vi "seatLeakageTest.vi"(7 "LabVIEW Web Service Request":refnum<class "Web Request.lvclass">, 10 "testPressure":dbl, 11 "time":dbl) -> (2 "startingPressure":dbl format="%#_2g", 3 "finalPressure":dbl)   [LabVIEW 2015]
uses:
  <vilib>/wsapi/Web Request.lvclass
  <vilib>/Waveform/WDTOps.llb/WDT Append Waveforms DBL.vi
panel:
  in  "Stop (Pressure Reading)":bool
  out "data":waveform(dbl)[](graph)
  out "timer":dbl
  in  "Stop timer":bool
  in  "Start timer":bool
  out "value":string
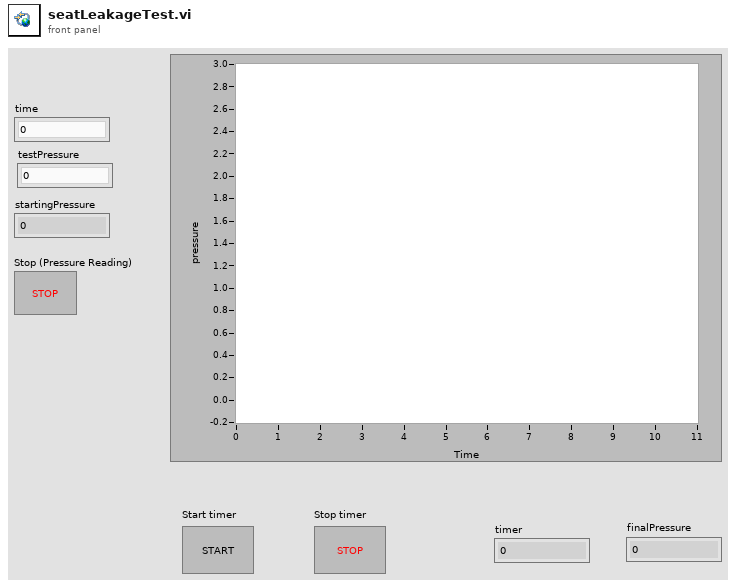
[diagram p1: front panel]
types:
  T1 = typedef "imagedata.ctl" = cluster{"image type":i32, "image depth":i32, "image":u8[], "mask":u8[], "colors":u32[], "Rectangle":cluster{"left":i16, "top":i16, "right":i16, "bottom":i16}}
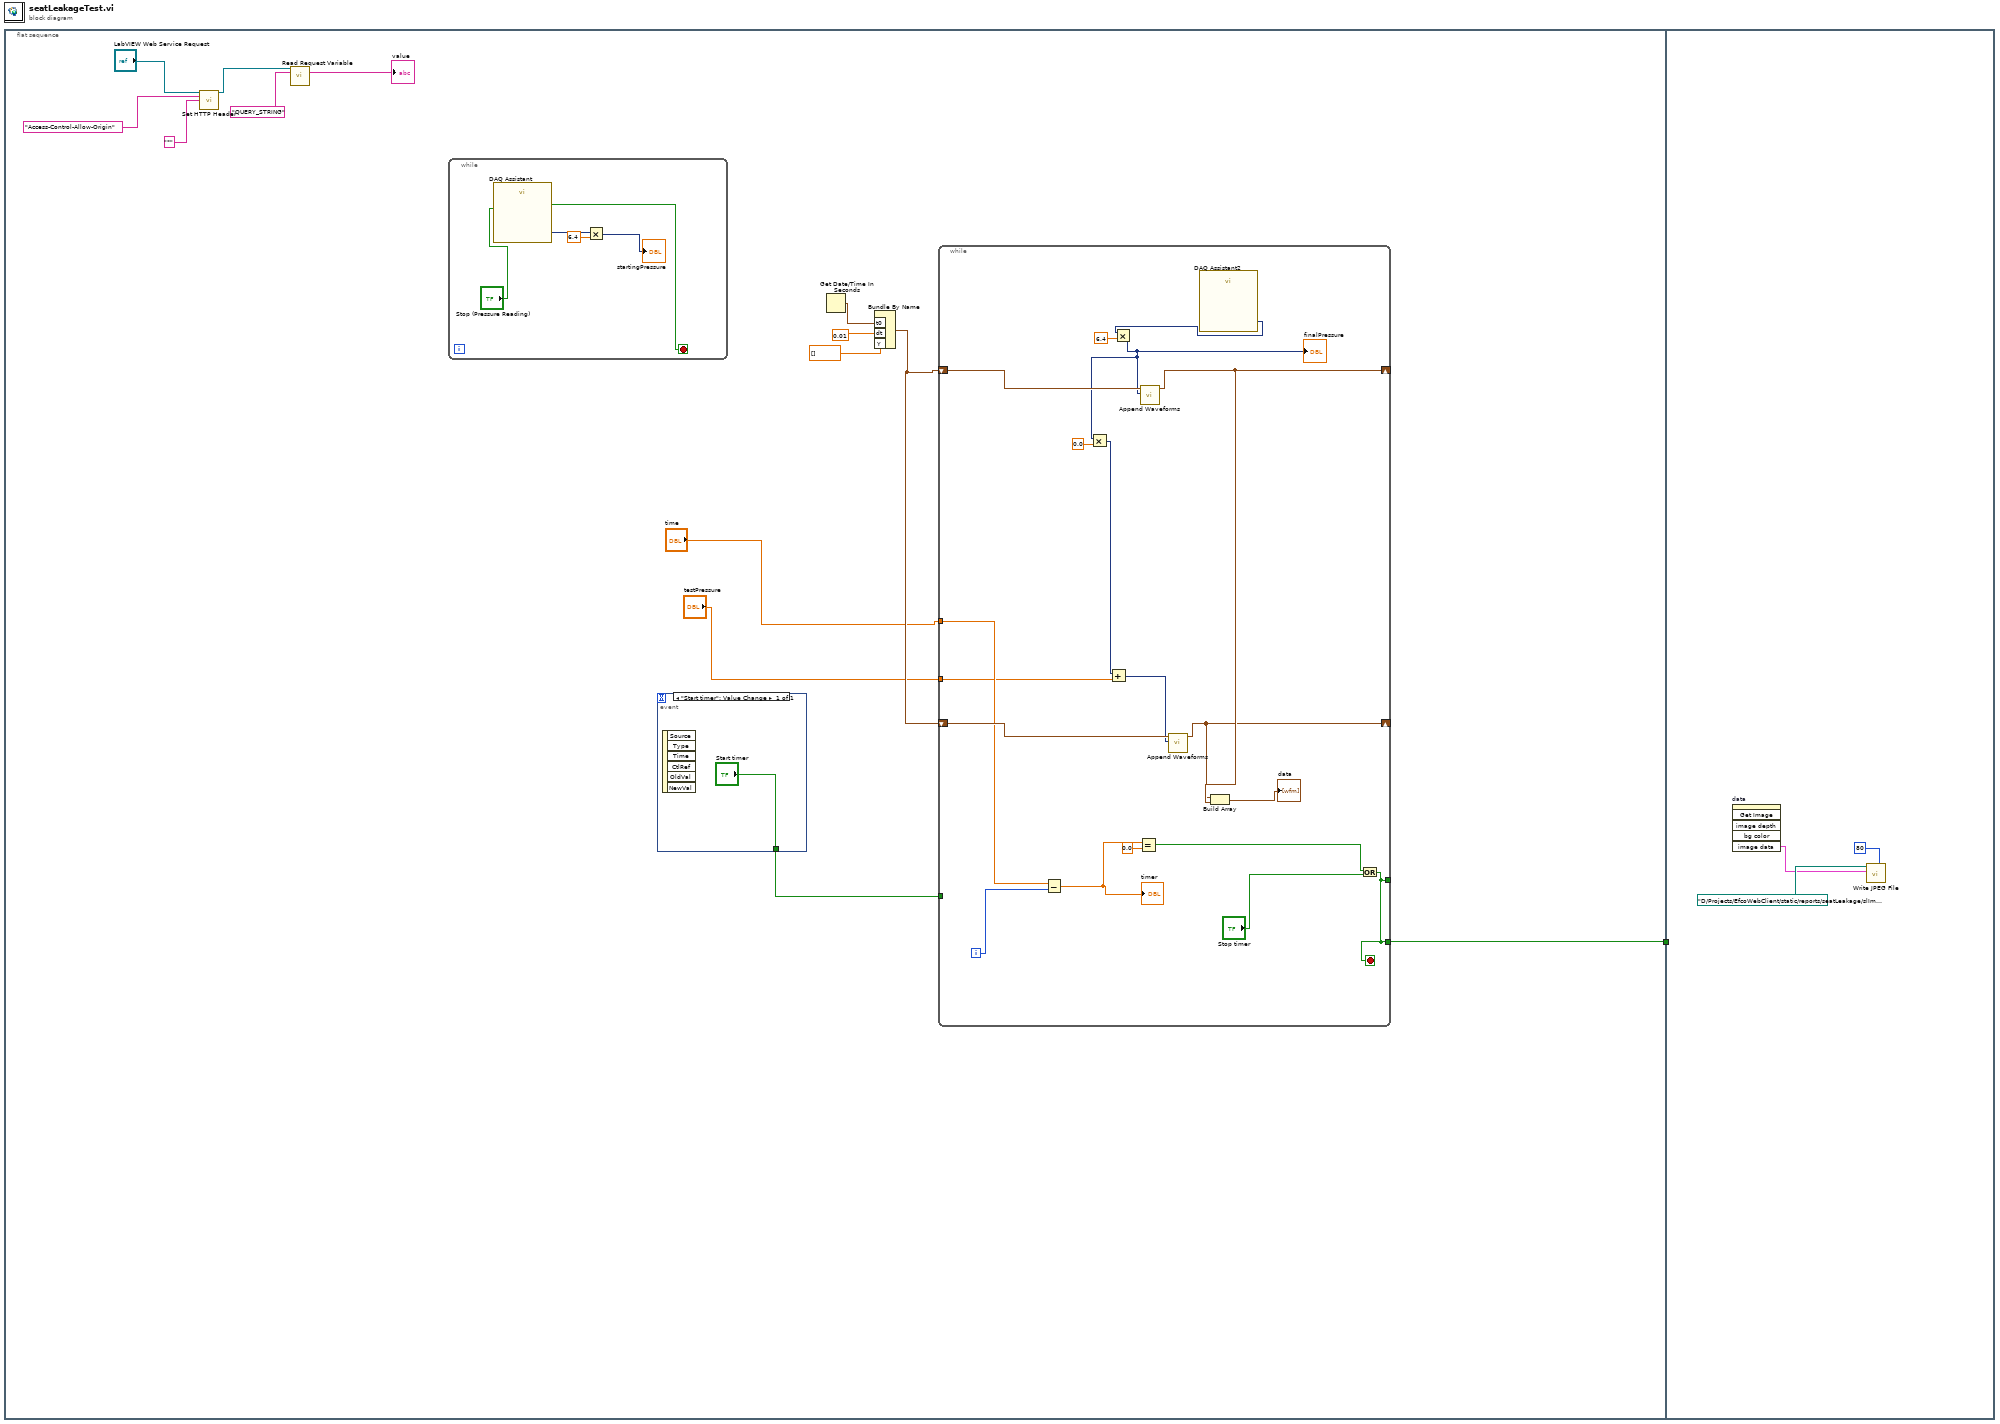
[diagram p0: block diagram]
diagram:
  n1 = flat-sequence {
    tunnel: [w8] -> w1
    tunnel: w1 -> [_]
    frame #0 {
      n2 = call <vilib>:"Set HTTP Header.vi"("LabVIEW Web Service Request"="LabVIEW Web Service Request", "header"="Access-Control-Allow-Origin", "header value"="*") -> ("LabVIEW Web Service Request out"=w4:refnum<class "Web Request.lvclass">)  [unwired: 11 in, 1 out]
      n3 = call <vilib>:"Read Request Variable.vi"("LabVIEW Web Service Request"=w4, "variable name"="QUERY_STRING") -> ("value"=→"value":string)  [unwired: 11 in, 2 out]
      n4 = while {
        stop <- w36 stop-if-true
        n5 = call "DAQ Assistant"("stop (F)"="Stop (Pressure Reading)") -> ("data"=w40:dynamicdata, "stopped"=w36:bool)  [unwired: 15 in, 2 out]
        n6 = Multiply(x=w40, y=6.4) -> (x*y=→"startingPressure":dynamicdata)
      }
      n7 = event shown="[0] \"Start timer\": Value Change" {
        selector: _ -> [_]
        dyn-events: _ -> [_]
        timeout: _ -> [_]
        tunnel: ["Start timer"] -> w12
        event "Start timer": Value Change {
          n8 = event-data() -> ()  [unwired: 1 in, 6 out]
        }
      }
      n9 = Get Date/Time In Seconds() -> (seconds since 1Jan1904=w15:timestamp)
      n10 = Bundle By Name("t0"=w15, "dt"=0.01, "Y"=dbl[] []) -> (w11:waveform(dbl))  [unwired: 1 in]
      n11 = while {
        shift-right: [w29] -> _
        shift-left: w11 -> [w35]
        tunnel: "time" -> [w25]
        shift-right: [w28] -> _
        shift-left: w11 -> [w33]
        tunnel: w12 -> [_]
        tunnel: "testPressure" -> [w19]
        tunnel: [w17] -> w8
        tunnel: [w17] -> _
        i -> [w26]
        stop <- w17 stop-if-true
        n12 = Subtract(x=w25, y=w26) -> (x-y=w24:dbl)
        "timer" <- w24
        n13 = Equal?(x=w24, y=0.0) -> (x = y?=w22:bool)
        n14 = call "DAQ Assistant2"() -> ("data"=w27:dynamicdata)  [unwired: 16 in, 3 out]
        n15 = Multiply(x=w27, y=6.4) -> (x*y=w32:dynamicdata)
        "finalPressure" <- w32
        n16 = Multiply(x=w32, y=0.0) -> (x*y=w30:dynamicdata)
        n17 = Add(x=w30, y=w19) -> (x+y=w20:dynamicdata)
        n18 = call-poly <vilib>:"Append Waveforms.vi"("waveform B"=w32, "waveform A"=w35) -> ("waveform out"=w29:waveform(dbl))  [unwired: 8 in, 1 out]
        n19 = call-poly <vilib>:"Append Waveforms.vi"("waveform B"=w20, "waveform A"=w33) -> ("waveform out"=w28:waveform(dbl))  [unwired: 8 in, 1 out]
        n20 = Build Array(w28, w29) -> (→"data":waveform(dbl)[])
        n21 = Or(x=w22, y="Stop timer") -> (x .or. y?=w17:bool)
      }
    }
    frame #1 {
      n22 = invoke on="data" class="WFGraph (strict)" method="Get Image"() -> ("image data"=w42:T1)  [unwired: 6 in, 5 out]
      n23 = call <vilib>:"Write JPEG File.vi"("quality (80)"=80, "image data"=w42, "path to JPEG file"=path "D:/Projects/EfcoWebClient/static/reports/seatLeakage/slImg.jpg") -> ()  [unwired: 7 in, 2 out]
    }
  }
